vi "rsscope_core_global.vi"() -> ()   [LabVIEW 2014] (continued)
"Supported Models"="RTO|RTP", "Instrument Options"="K72", "Flags"=0, "Help"="Sets the completer ID to be searched for in the transaction layer type.\n\nAvailable Repeated Capabilities:\nNone\n\nRemote-control command(s):\nSEARch:TRIGger:PCIE:TLP:CPID"}, {"Level"=4, "Class Only"=TRUE, "Identifier"="", "Descriptive Name"="DLLP", "Data Type"=0, "Command"="", "Access"=0, "Range Table"="", "Read Callback"="", "Write Callback"="", "Supported Models"="", "Instrument Options"="", "Flags"=0, "Help"="Configures data link layer search."}, {"Level"=5, "Class Only"=FALSE, "Identifier"="RSSCOPE_ATTR_PCIE_SEARCH_DLLP", "Descriptive Name"="PCIe Search DLLP", "Data Type"=0, "Command"="SEAR:TRIG:PCIE:DLLP:TYPE", "Access"=2, "Range Table"="RsScope_rngPCIeDLLP", "Read Callback"="rsscope_FormatSearchNameInt32_ReadCallback.vi", "Write Callback"="rsscope_FormatSearchNameInt32_WriteCallback.vi", "Supported Models"="RTO|RTP", "Instrument Options"="K72", "Flags"=0, "Help"="Sets the DLLP t type to be searched for, for the data link layer.\n\nAvailable Repeated Capabilities:\nNone\n\nRemote-control command(s):\nSEARch:TRIGger:PCIE:DLLP:TYPE"}, {"Level"=5, "Class Only"=FALSE, "Identifier"="RSSCOPE_ATTR_PCIE_SEARCH_DLLP_MR_TYPE", "Descriptive Name"="PCIe Search DLLP MR Type", "Data Type"=0, "Command"="SEAR:TRIG:PCIE:DLLP:MULT:TYPE", "Access"=2, "Range Table"="RsScope_rngPCIeDLLPMRType", "Read Callback"="rsscope_FormatSearchNameInt32_ReadCallback.vi", "Write Callback"="rsscope_FormatSearchNameInt32_WriteCallback.vi", "Supported Models"="RTO|RTP", "Instrument Options"="K72", "Flags"=0, "Help"="Sets the multi-root type to be searched for, for the data link layer.\n\nAvailable Repeated Capabilities:\nNone\n\nRemote-control command(s):\nSEARch:TRIGger:PCIE:DLLP:MULT:TYPE"}, {"Level"=5, "Class Only"=FALSE, "Identifier"="RSSCOPE_ATTR_PCIE_SEARCH_DLLP_MR_INIT_PHASE", "Descriptive Name"="PCIe Search DLLP MR Init Phase", "Data Type"=0, "Command"="SEAR:TRIG:PCIE:DLLP:MULT:PHAS", "Access"=2, "Range Table"="RsScope_rngPCIeState", "Read Callback"="rsscope_FormatSearchNameInt32_ReadCallback.vi", "Write Callback"="rsscope_FormatSearchNameInt32_WriteCallback.vi", "Supported Models"="RTO|RTP", "Instrument Options"="K72", "Flags"=0, "Help"="Sets the phase state to be searched for, for the data link layer.\n\nAvailable Repeated Capabilities:\nNone\n\nRemote-control command(s):\nSEARch:TRIGger:PCIE:DLLP:MULT:PHAS"}, {"Level"=5, "Class Only"=FALSE, "Identifier"="RSSCOPE_ATTR_PCIE_SEARCH_DLLP_MR_INIT_VH_FC", "Descriptive Name"="PCIe Search DLLP MR Init VH FC", "Data Type"=0, "Command"="SEAR:TRIG:PCIE:DLLP:MULT:VHFC", "Access"=2, "Range Table"="RsScope_rngPCIeState", "Read Callback"="rsscope_FormatSearchNameInt32_ReadCallback.vi", "Write Callback"="rsscope_FormatSearchNameInt32_WriteCallback.vi", "Supported Models"="RTO|RTP", "Instrument Options"="K72", "Flags"=0, "Help"="Sets the virtual hierarchies flow control presence state to be searched for, for the data link layer.\n\nAvailable Repeated Capabilities:\nNone\n\nRemote-control command(s):\nSEARch:TRIGger:PCIE:DLLP:MULT:VHFC"}, {"Level"=5, "Class Only"=FALSE, "Identifier"="RSSCOPE_ATTR_PCIE_SEARCH_DLLP_MR_INIT_MIXED_TYPE", "Descriptive Name"="PCIe Search DLLP MR Init Mixed Type", "Data Type"=0, "Command"="SEAR:TRIG:PCIE:DLLP:MULT:MIXT", "Access"=2, "Range Table"="RsScope_rngPCIeState", "Read Callback"="rsscope_FormatSearchNameInt32_ReadCallback.vi", "Write Callback"="rsscope_FormatSearchNameInt32_WriteCallback.vi", "Supported Models"="RTO|RTP", "Instrument Options"="K72", "Flags"=0, "Help"="Sets the mixed type presence state to be searched for, for the data link layer.\n\nAvailable Repeated Capabilities:\nNone\n\nRemote-control command(s):\nSEARch:TRIGger:PCIE:DLLP:MULT:MIXT"}, {"Level"=5, "Class Only"=FALSE, "Identifier"="RSSCOPE_ATTR_PCIE_SEARCH_DLLP_MR_INIT_AUTHORIZED", "Descriptive Name"="PCIe Search DLLP MR Init Authorized", "Data Type"=0, "Command"="SEAR:TRIG:PCIE:DLLP:MULT:AUTH", "Access"=2, "Range Table"="RsScope_rngPCIeState", "Read Callback"="rsscope_FormatSearchNameInt32_ReadCallback.vi", "Write Callback"="rsscope_FormatSearchNameInt32_WriteCallback.vi", "Supported Models"="RTO|RTP", "Instrument Options"="K72", "Flags"=0, "Help"="Sets the authorized presence state to be searched for, for the data link layer.\n\nAvailable Repeated Capabilities:\nNone\n\nRemote-control command(s):\nSEARch:TRIGger:PCIE:DLLP:MULT:AUTH"}, {"Level"=5, "Class Only"=FALSE, "Identifier"="RSSCOPE_ATTR_PCIE_SEARCH_DLLP_MR_INIT_DEVICE_PORT_TYPE", "Descriptive Name"="PCIe Search DLLP MR Init Device Port Type", "Data Type"=0, "Command"="SEAR:TRIG:PCIE:DLLP:MULT:DVPT", "Access"=2, "Range Table"="RsScope_rngPCIeDevicePortType", "Read Callback"="rsscope_FormatSearchNameInt32_ReadCallback.vi", "Write Callback"="rsscope_FormatSearchNameInt32_WriteCallback.vi", "Supported Models"="RTO|RTP", "Instrument Options"="K72", "Flags"=0, "Help"="Sets the device/port type to be searched for, for the data link layer.\n\nAvailable Repeated Capabilities:\nNone\n\nRemote-control command(s):\nSEARch:TRIGger:PCIE:DLLP:MULT:DVPT"}, {"Level"=5, "Class Only"=FALSE, "Identifier"="RSSCOPE_ATTR_PCIE_SEARCH_DLLP_MR_VL_NUMBER", "Descriptive Name"="PCIe Search DLLP MR VL Number", "Data Type"=0, "Command"="SEAR:TRIG:PCIE:DLLP:MULT:VLNR", "Access"=2, "Range Table"="RsScope_rngPCIeVLNumber", "Read Callback"="rsscope_FormatSearchNameInt32_ReadCallback.vi", "Write Callback"="rsscope_FormatSearchNameInt32_WriteCallback.vi", "Supported Models"="RTO|RTP", "Instrument Options"="K72", "Flags"=0, "Help"="Sets the virtual link (VL) number to be searched for, for the data link layer.\n\nAvailable Repeated Capabilities:\nNone\n\nRemote-control command(s):\nSEARch:TRIGger:PCIE:DLLP:MULT:VLNR"}, {"Level"=5, "Class Only"=FALSE, "Identifier"="RSSCOPE_ATTR_PCIE_SEARCH_DLLP_MR_VH_ABSENT", "Descriptive Name"="PCIe Search DLLP MR VH Absent", "Data Type"=0, "Command"="SEAR:TRIG:PCIE:DLLP:MULT:HABS", "Access"=2, "Range Table"="RsScope_rngPCIeState", "Read Callback"="rsscope_FormatSearchNameInt32_ReadCallback.vi", "Write Callback"="rsscope_FormatSearchNameInt32_WriteCallback.vi", "Supported Models"="RTO|RTP", "Instrument Options"="K72", "Flags"=0, "Help"="Sets the state of the absent virtual hieararchies (VH) to be searched for, for the data link layer.\n\nAvailable Repeated Capabilities:\nNone\n\nRemote-control command(s):\nSEARch:TRIGger:PCIE:DLLP:MULT:HABS"}, {"Level"=5, "Class Only"=FALSE, "Identifier"="RSSCOPE_ATTR_PCIE_SEARCH_DLLP_MR_TLP_TYPE", "Descriptive Name"="PCIe Search DLLP MR TLP Type", "Data Type"=0, "Command"="SEAR:TRIG:PCIE:DLLP:MULT:TLPT", "Access"=2, "Range Table"="RsScope_rngPCIeDLLPMRTLPType", "Read Callback"="rsscope_FormatSearchNameInt32_ReadCallback.vi", "Write Callback"="rsscope_FormatSearchNameInt32_WriteCallback.vi", "Supported Models"="RTO|RTP", "Instrument Options"="K72", "Flags"=0, "Help"="Sets the multi-root type to be searched for, for the data link layer.\n\nAvailable Repeated Capabilities:\nNone\n\nRemote-control command(s):\nSEARch:TRIGger:PCIE:DLLP:MULT:TLPT"}, {"Level"=5, "Class Only"=FALSE, "Identifier"="RSSCOPE_ATTR_PCIE_SEARCH_DLLP_MR_CREDIT_TYPE", "Descriptive Name"="PCIe Search DLLP MR Credit Type", "Data Type"=0, "Command"="SEAR:TRIG:PCIE:DLLP:MULT:CRET", "Access"=2, "Range Table"="RsScope_rngPCIeDLLPMRCreditType", "Read Callback"="rsscope_FormatSearchNameInt32_ReadCallback.vi", "Write Callback"="rsscope_FormatSearchNameInt32_WriteCallback.vi", "Supported Models"="RTO|RTP", "Instrument Options"="", "Flags"=0, "Help"="Sets the credit type to be searched for, for the data link layer.\n\nAvailable Repeated Capabilities:\nNone\n\nRemote-control command(s):\nSEARch:TRIGger:PCIE:DLLP:MULT:CRET"}, {"Level"=5, "Class Only"=FALSE, "Identifier"="RSSCOPE_ATTR_PCIE_SEARCH_DLLP_MR_A", "Descriptive Name"="PCIe Search DLLP MR A", "Data Type"=0, "Command"="SEAR:TRIG:PCIE:DLLP:MULT:RESA", "Access"=2, "Range Table"="RsScope_rngPCIeTriggerDLLPMRA", "Read Callback"="rsscope_FormatSearchNameInt32_ReadCallback.vi", "Write Callback"="rsscope_FormatSearchNameInt32_WriteCallback.vi", "Supported Models"="RTO|RTP", "Instrument Options"="K72", "Flags"=0, "Help"="Sets the on the value of the A bit to be searched for, for the data link layer.\n\nAvailable Repeated Capabilities:\nNone\n\nRemote-control command(s):\nSEARch:TRIGger:PCIE:DLLP:MULT:RESA"}, {"Level"=5, "Class Only"=FALSE, "Identifier"="RSSCOPE_ATTR_PCIE_SEARCH_DLLP_MR_VH_GROUP", "Descriptive Name"="PCIe Search DLLP MR VH Group", "Data Type"=0, "Command"="SEAR:TRIG:PCIE:DLLP:MULT:VHGR", "Access"=2, "Range Table"="RsScope_rngPCIeDLLPVHGroup", "Read Callback"="rsscope_FormatSearchNameInt32_ReadCallback.vi", "Write Callback"="rsscope_FormatSearchNameInt32_WriteCallback.vi", "Supported Models"="RTO|RTP", "Instrument Options"="K72", "Flags"=0, "Help"="Sets the virtual hierarchies group to be searched for, for the data link layer.\n\nAvailable Repeated Capabilities:\nNone\n\nRemote-control command(s):\nSEARch:TRIGger:PCIE:DLLP:MULT:VHGR"}, {"Level"=5, "Class Only"=FALSE, "Identifier"="RSSCOPE_ATTR_PCIE_SEARCH_DLLP_SEQUENCE", "Descriptive Name"="PCIe Search DLLP Sequence", "Data Type"=2, "Command"="SEAR:TRIG:PCIE:DLLP:SEQ", "Access"=2, "Range Table"="", "Read Callback"="rsscope_FormatSearchNameString_ReadCallback.vi", "Write Callback"="rsscope_FormatSearchNameString_WriteCallback.vi", "Supported Models"="RTO|RTP", "Instrument Options"="K72", "Flags"=0, "Help"="Sets the sequence field, indicating what TLPs are affected by the ACK/NAK, to be searched for, for the data link layer.\n\nAvailable Repeated Capabilities:\nNone\n\nRemote-control command(s):\nSEARch:TRIGger:PCIE:DLLP:SEQ"}, {"Level"=5, "Class Only"=FALSE, "Identifier"="RSSCOPE_ATTR_PCIE_SEARCH_DLLP_FC_CREDIT_TYPE", "Descriptive Name"="PCIe Search DLLP FC Credit Type", "Data Type"=0, "Command"="SEAR:TRIG:PCIE:DLLP:FCTL:CRET", "Access"=2, "Range Table"="RsScope_rngPCIeDLLPFCCreditType", "Read Callback"="rsscope_FormatSearchNameInt32_ReadCallback.vi", "Write Callback"="rsscope_FormatSearchNameInt32_WriteCallback.vi", "Supported Models"="RTO|RTP", "Instrument Options"="K72", "Flags"=0, "Help"="Sets credit type value to be searched for, for the data link layer.\n\nAvailable Repeated Capabilities:\nNone\n\nRemote-control command(s):\nSEARch:TRIGger:PCIE:DLLP:FCTL:CRET"}, {"Level"=5, "Class Only"=FALSE, "Identifier"="RSSCOPE_ATTR_PCIE_SEARCH_DLLP_FC_VC_ID", "Descriptive Name"="PCIe Search DLLP FC VC ID", "Data Type"=0, "Command"="SEAR:TRIG:PCIE:DLLP:FCTL:VCID", "Access"=2, "Range Table"="RsScope_rngPCIeDLLPVCID", "Read Callback"="rsscope_FormatSearchNameInt32_ReadCallback.vi", "Write Callback"="rsscope_FormatSearchNameInt32_WriteCallback.vi", "Supported Models"="RTO|RTP", "Instrument Options"="K72", "Flags"=0, "Help"="Sets the virtual channel ID to be searched for, for the data link layer.\n\nAvailable Repeated Capabilities:\nNone\n\nRemote-control command(s):\nSEARch:TRIGger:PCIE:DLLP:FCTL:VCID"}, {"Level"=5, "Class Only"=FALSE, "Identifier"="RSSCOPE_ATTR_PCIE_SEARCH_DLLP_PM_TYPE", "Descriptive Name"="PCIe Search DLLP PM Type", "Data Type"=0, "Command"="SEAR:TRIG:PCIE:DLLP:POWM", "Access"=2, "Range Table"="RsScope_rngPCIeDLLPPMType", "Read Callback"="rsscope_FormatSearchNameInt32_ReadCallback.vi", "Write Callback"="rsscope_FormatSearchNameInt32_WriteCallback.vi", "Supported Models"="RTO|RTP", "Instrument Options"="K72", "Flags"=0, "Help"="Sets the power management type to be searched for, for the data link layer.\n\nAvailable Repeated Capabilities:\nNone\n\nRemote-control command(s):\nSEARch:TRIGger:PCIE:DLLP:POWM"}, {"Level"=5, "Class Only"=FALSE, "Identifier"="RSSCOPE_ATTR_PCIE_SEARCH_DLLP_VENDOR_PATTERN", "Descriptive Name"="PCIe Search DLLP Vendor Pattern", "Data Type"=2, "Command"="SEAR:TRIG:PCIE:DLLP:VPAT", "Access"=2, "Range Table"="", "Read Callback"="rsscope_FormatSearchNameString_ReadCallback.vi", "Write Callback"="rsscope_FormatSearchNameString_WriteCallback.vi", "Supported Models"="RTO|RTP", "Instrument Options"="K72", "Flags"=0, "Help"="Sets the vendor pattern to be searched for, for the data link layer.\n\nAvailable Repeated Capabilities:\nNone\n\nRemote-control command(s):\nSEARch:TRIGger:PCIE:DLLP:VPAT"}, {"Level"=4, "Class Only"=TRUE, "Identifier"="", "Descriptive Name"="Ordered Sets", "Data Type"=0, "Command"="", "Access"=0, "Range Table"="", "Read Callback"="", "Write Callback"="", "Supported Models"="", "Instrument Options"="", "Flags"=0, "Help"="Configures the search on a defined ordered set."}, {"Level"=5, "Class Only"=FALSE, "Identifier"="RSSCOPE_ATTR_PCIE_SEARCH_OSET_TRAINING_SEQUENCE_1", "Descriptive Name"="PCIe Search OSET Training Sequence 1", "Data Type"=3, "Command"="SEAR:TRIG:PCIE:OSET:TSON", "Access"=2, "Range Table"="", "Read Callback"="rsscope_FormatSearchNameBoolean_ReadCallback.vi", "Write Callback"="rsscope_FormatSearchNameBoolean_WriteCallback.vi", "Supported Models"="RTO|RTP", "Instrument Options"="K72", "Flags"=0, "Help"="Enables searching for training sequence 1 ordered sets.\n\nAvailable Repeated Capabilities:\nNone\n\nRemote-control command(s):\nSEARch:TRIGger:PCIE:OSET:TSONe"}, {"Level"=5, "Class Only"=FALSE, "Identifier"="RSSCOPE_ATTR_PCIE_SEARCH_OSET_TRAINING_SEQUENCE_2", "Descriptive Name"="PCIe Search OSET Training Sequence 2", "Data Type"=3, "Command"="SEARch:TRIGger:PCIE:OSET:TSTWo", "Access"=2, "Range Table"="", "Read Callback"="rsscope_FormatSearchNameBoolean_ReadCallback.vi", "Write Callback"="rsscope_FormatSearchNameBoolean_WriteCallback.vi", "Supported Models"="RTO|RTP", "Instrument Options"="K72", "Flags"=0, "Help"="Enables searching for training sequence 2 ordered sets.\n\nAvailable Repeated Capabilities:\nNone\n\nRemote-control command(s):\nSEARch:TRIGger:PCIE:OSET:TSTWo"}, {"Level"=5, "Class Only"=FALSE, "Identifier"="RSSCOPE_ATTR_PCIE_SEARCH_OSET_FAST_TRAINING_SEQUENCE", "Descriptive Name"="PCIe Search OSET Fast Training Sequence", "Data Type"=3, "Command"="SEAR:TRIG:PCIE:OSET:FTS", "Access"=2, "Range Table"="", "Read Callback"="rsscope_FormatSearchNameBoolean_ReadCallback.vi", "Write Callback"="rsscope_FormatSearchNameBoolean_WriteCallback.vi", "Supported Models"="RTO|RTP", "Instrument Options"="K72", "Flags"=0, "Help"="Enables searching for fast training sequence ordered sets.\n\nAvailable Repeated Capabilities:\nNone\n\nRemote-control command(s):\nSEARch:TRIGger:PCIE:OSET:FTS"}, {"Level"=5, "Class Only"=FALSE, "Identifier"="RSSCOPE_ATTR_PCIE_SEARCH_OSET_EIDL", "Descriptive Name"="PCIe Search OSET Electrical Idle", "Data Type"=3, "Command"="SEAR:TRIG:PCIE:OSET:EIDL", "Access"=2, "Range Table"="", "Read Callback"="rsscope_FormatSearchNameBoolean_ReadCallback.vi", "Write Callback"="rsscope_FormatSearchNameBoolean_WriteCallback.vi", "Supported Models"="RTO|RTP", "Instrument Options"="K72", "Flags"=0, "Help"="Enables searching for electrical idle ordered sets.\n\nAvailable Repeated Capabilities:\nNone\n\nRemote-control command(s):\nSEARch:TRIGger:PCIE:OSET:EIDL"}, {"Level"=5, "Class Only"=FALSE, "Identifier"="RSSCOPE_ATTR_PCIE_SEARCH_OSET_EIDE", "Descriptive Name"="PCIe Search OSET Electrical Idle Exit", "Data Type"=3, "Command"="SEAR:TRIG:PCIE:OSET:EIDE", "Access"=2, "Range Table"="", "Read Callback"="rsscope_FormatSearchNameBoolean_ReadCallback.vi", "Write Callback"="rsscope_FormatSearchNameBoolean_WriteCallback.vi", "Supported Models"="RTO|RTP", "Instrument Options"="K72", "Flags"=0, "Help"="Enables searching for electrical idle exit ordered sets.\n\nAvailable Repeated Capabilities:\nNone\n\nRemote-control command(s):\nSEARch:TRIGger:PCIE:OSET:EIDE"}, {"Level"=5, "Class Only"=FALSE, "Identifier"="RSSCOPE_ATTR_PCIE_SEARCH_OSET_SKP", "Descriptive Name"="PCIe Search OSET SKP", "Data Type"=3, "Command"="SEAR:TRIG:PCIE:OSET:SKIP", "Access"=2, "Range Table"="", "Read Callback"="rsscope_FormatSearchNameBoolean_ReadCallback.vi", "Write Callback"="rsscope_FormatSearchNameBoolean_WriteCallback.vi", "Supported Models"="RTO|RTP", "Instrument Options"="K72", "Flags"=0, "Help"="Enables searching for SKP ordered sets.\n\nAvailable Repeated Capabilities:\nNone\n\nRemote-control command(s):\nSEARch:TRIGger:PCIE:OSET:SKIP"}, {"Level"=5, "Class Only"=FALSE, "Identifier"="RSSCOPE_ATTR_PCIE_SEARCH_OSET_COMP", "Descriptive Name"="PCIe Search OSET Compliance Pattern", "Data Type"=3, "Command"="SEAR:TRIG:PCIE:OSET:COMP", "Access"=2, "Range Table"="", "Read Callback"="rsscope_FormatSearchNameBoolean_ReadCallback.vi", "Write Callback"="rsscope_FormatSearchNameBoolean_WriteCallback.vi", "Supported Models"="RTO|RTP", "Instrument Options"="K72", "Flags"=0, "Help"="Enables searching forcompliance pattern ordered sets.\n\nAvailable Repeated Capabilities:\nNone\n\nRemote-control command(s):\nSEARch:TRIGger:PCIE:OSET:COMP"}, {"Level"=5, "Class Only"=FALSE, "Identifier"="RSSCOPE_ATTR_PCIE_SEARCH_OSET_START_OF_DATA_SEQUENCE", "Descriptive Name"="PCIe Search OSET Start Of Data Sequence", "Data Type"=3, "Command"="SEAR:TRIG:PCIE:OSET:SDS", "Access"=2, "Range Table"="", "Read Callback"="rsscope_FormatSearchNameBoolean_ReadCallback.vi", "Write Callback"="rsscope_FormatSearchNameBoolean_WriteCallback.vi", "Supported Models"="RTO|RTP", "Instrument Options"="K72", "Flags"=0, "Help"="Enables searching for a start of data sequence order set.\n\nAvailable Repeated Capabilities:\nNone\n\nRemote-control command(s):\nSEARch:TRIGger:PCIE:OSET:SDS"}, {"Level"=4, "Class Only"=TRUE, "Identifier"="", "Descriptive Name"="Error Condition", "Data Type"=0, "Command"="", "Access"=0, "Range Table"="", "Read Callback"="", "Write Callback"="", "Supported Models"="", "Instrument Options"="", "Flags"=0, "Help"="Search on enabled error condition."}, {"Level"=5, "Class Only"=FALSE, "Identifier"="RSSCOPE_ATTR_PCIE_SEARCH_ERRC_CRC16", "Descriptive Name"="PCIe Search ERRC CRC16 Error", "Data Type"=3, "Command"="SEAR:TRIG:PCIE:ERRC:CRC", "Access"=2, "Range Table"="", "Read Callback"="rsscope_FormatSearchNameBoolean_ReadCallback.vi", "Write Callback"="rsscope_FormatSearchNameBoolean_WriteCallback.vi", "Supported Models"="RTO|RTP", "Instrument Options"="K72", "Flags"=0, "Help"="Enables searching for 16-bit cyclic redundancy check (CRC) errors.\n\nAvailable Repeated Capabilities:\nNone\n\nRemote-control command(s):\nSEARch:TRIGger:PCIE:ERRC:CRC"}, {"Level"=5, "Class Only"=FALSE, "Identifier"="RSSCOPE_ATTR_PCIE_SEARCH_ERRC_LCRC", "Descriptive Name"="PCIe Search ERRC LCRC Error", "Data Type"=3, "Command"="SEAR:TRIG:PCIE:ERRC:LCRC", "Access"=2, "Range Table"="", "Read Callback"="rsscope_FormatSearchNameBoolean_ReadCallback.vi", "Write Callback"="rsscope_FormatSearchNameBoolean_WriteCallback.vi", "Supported Models"="RTO|RTP", "Instrument Options"="K72", "Flags"=0, "Help"="Enables searching for link cyclic redundancy check (LCRC) errors.\n\nAvailable Repeated Capabilities:\nNone\n\nRemote-control command(s):\nSEARch:TRIGger:PCIE:ERRC:LCRC"}, {"Level"=5, "Class Only"=FALSE, "Identifier"="RSSCOPE_ATTR_PCIE_SEARCH_ERRC_ECRC", "Descriptive Name"="PCIe Search ERRC ECRC Error", "Data Type"=3, "Command"="SEAR:TRIG:PCIE:ERRC:ECRC", "Access"=2, "Range Table"="", "Read Callback"="rsscope_FormatSearchNameBoolean_ReadCallback.vi", "Write Callback"="rsscope_FormatSearchNameBoolean_WriteCallback.vi", "Supported Models"="RTO|RTP", "Instrument Options"="K72", "Flags"=0, "Help"="Enables searching for end-to-end cyclic redundancy checksum (ECRC) errors.\n\nAvailable Repeated Capabilities:\nNone\n\nRemote-control command(s):\nSEARch:TRIGger:PCIE:ERRC:ECRC"}, {"Level"=5, "Class Only"=FALSE, "Identifier"="RSSCOPE_ATTR_PCIE_SEARCH_ERRC_INVALID_SYMBOL", "Descriptive Name"="PCIe Search ERRC Invalid Symbol", "Data Type"=3, "Command"="SEAR:TRIG:PCIE:ERRC:INVP", "Access"=2, "Range Table"="", "Read Callback"="rsscope_FormatSearchNameBoolean_ReadCallback.vi", "Write Callback"="rsscope_FormatSearchNameBoolean_WriteCallback.vi", "Supported Models"="RTO|RTP", "Instrument Options"="K72", "Flags"=0, "Help"="Enables searching for invalid symbol errors.\n\nAvailable Repeated Capabilities:\nNone\n\nRemote-control command(s):\nSEARch:TRIGger:PCIE:ERRC:INVP"}, {"Level"=5, "Class Only"=FALSE, "Identifier"="RSSCOPE_ATTR_PCIE_SEARCH_ERRC_DISP", "Descriptive Name"="PCIe Search ERRC Disparity Error", "Data Type"=3, "Command"="SEAR:TRIG:PCIE:ERRC:DISP", "Access"=2, "Range Table"="", "Read Callback"="rsscope_FormatSearchNameBoolean_ReadCallback.vi", "Write Callback"="rsscope_FormatSearchNameBoolean_WriteCallback.vi", "Supported Models"="RTO|RTP", "Instrument Options"="K72", "Flags"=0, "Help"="Enables searching for disparity errors.\n\nAvailable Repeated Capabilities:\nNone\n\nRemote-control command(s):\nSEARch:TRIGger:PCIE:ERRC:DISP"}, {"Level"=5, "Class Only"=FALSE, "Identifier"="RSSCOPE_ATTR_PCIE_SEARCH_ERRC_LENGTH_ERROR", "Descriptive Name"="PCIe Search ERRC Length Error", "Data Type"=3, "Command"="SEAR:TRIG:PCIE:ERRC:LENG", "Access"=2, "Range Table"="", "Read Callback"="rsscope_FormatSearchNameBoolean_ReadCallback.vi", "Write Callback"="rsscope_FormatSearchNameBoolean_WriteCallback.vi", "Supported Models"="RTO|RTP", "Instrument Options"="K72", "Flags"=0, "Help"="Enables searching for length error.\n\nAvailable Repeated Capabilities:\nNone\n\nRemote-control command(s):\nSEARch:TRIGger:PCIE:ERRC:LENGth"}, {"Level"=5, "Class Only"=FALSE, "Identifier"="RSSCOPE_ATTR_PCIE_SEARCH_ERRC_MALFORMED_ERROR", "Descriptive Name"="PCIe Search ERRC Malformed Error", "Data Type"=3, "Command"="SEAR:TRIG:PCIE:ERRC:MALF", "Access"=2, "Range Table"="", "Read Callback"="rsscope_FormatSearchNameBoolean_ReadCallback.vi", "Write Callback"="rsscope_FormatSearchNameBoolean_WriteCallback.vi", "Supported Models"="RTO|RTP", "Instrument Options"="K72", "Flags"=0, "Help"="Searches for a malformed TLP: a TLP that violates specific TLP formation rules that are defined in the specification.\n\nAvailable Repeated Capabilities:\nNone\n\nRemote-control command(s):\nSEARch:TRIGger:PCIE:ERRC:MALFormed"}, {"Level"=5, "Class Only"=FALSE, "Identifier"="RSSCOPE_ATTR_PCIE_SEARCH_ERRC_MAX_END_PREFIX", "Descriptive Name"="PCIe Search ERRC Max End Prefix", "Data Type"=3, "Command"="SEAR:TRIG:PCIE:ERRC:MXPF", "Access"=2, "Range Table"="", "Read Callback"="rsscope_FormatSearchNameBoolean_ReadCallback.vi", "Write Callback"="rsscope_FormatSearchNameBoolean_WriteCallback.vi", "Supported Models"="RTO|RTP", "Instrument Options"="K72", "Flags"=0, "Help"="Enables searching for an end-end prefix error. The maximum number of permitted end-end TLP prefixes is 4.\n\nAvailable Repeated Capabilities:\nNone\n\nRemote-control command(s):\nSEARch:TRIGger:PCIE:ERRC:MXPFix"}, {"Level"=5, "Class Only"=FALSE, "Identifier"="RSSCOPE_ATTR_PCIE_SEARCH_ERRC_PREFIX_ORDER_ERROR", "Descriptive Name"="PCIe Search ERRC Prefix Order Error", "Data Type"=3, "Command"="SEAR:TRIG:PCIE:ERRC:PFOR", "Access"=2, "Range Table"="", "Read Callback"="rsscope_FormatSearchNameBoolean_ReadCallback.vi", "Write Callback"="rsscope_FormatSearchNameBoolean_WriteCallback.vi", "Supported Models"="RTO|RTP", "Instrument Options"="K72", "Flags"=0, "Help"="Enables searching for a wrong prefix order\n\nAvailable Repeated Capabilities:\nNone\n\nRemote-control command(s):\nSEARch:TRIGger:PCIE:ERRC:PFORder"}, {"Level"=5, "Class Only"=FALSE, "Identifier"="RSSCOPE_ATTR_PCIE_SEARCH_ERRC_SYNC_BIT", "Descriptive Name"="PCIe Search ERRC Sync Bit", "Data Type"=3, "Command"="SEAR:TRIG:PCIE:ERRC:SYCB", "Access"=2, "Range Table"="", "Read Callback"="rsscope_FormatSearchNameBoolean_ReadCallback.vi", "Write Callback"="rsscope_FormatSearchNameBoolean_WriteCallback.vi", "Supported Models"="RTO|RTP", "Instrument Options"="K72", "Flags"=0, "Help"="Enables searching for a sync bit\n\nAvailable Repeated Capabilities:\nNone\n\nRemote-control command(s):\nSEARch:TRIGger:PCIE:ERRC:SYCBit"}, {"Level"=5, "Class Only"=FALSE, "Identifier"="RSSCOPE_ATTR_PCIE_SEARCH_ERRC_UNKNOWN_PACKET", "Descriptive Name"="PCIe Search ERRC Unknown Packet", "Data Type"=3, "Command"="SEAR:TRIG:PCIE:ERRC:UKNP", "Access"=2, "Range Table"="", "Read Callback"="rsscope_FormatSearchNameBoolean_ReadCallback.vi", "Write Callback"="rsscope_FormatSearchNameBoolean_WriteCallback.vi", "Supported Models"="RTO|RTP", "Instrument Options"="K72", "Flags"=0, "Help"="Enables searching for an unknown packet.\n\nAvailable Repeated Capabilities:\nNone\n\nRemote-control command(s):\nSEARch:TRIGger:PCIE:ERRC:UKNP"}, {"Level"=5, "Class Only"=FALSE, "Identifier"="RSSCOPE_ATTR_PCIE_SEARCH_ERRC_VALUE_OUT_OF_RANGE", "Descriptive Name"="PCIe Search ERRC Value Out Of Range", "Data Type"=3, "Command"="SEAR:TRIG:PCIE:ERRC:VOOR", "Access"=2, "Range Table"="", "Read Callback"="rsscope_FormatSearchNameBoolean_ReadCallback.vi", "Write Callback"="rsscope_FormatSearchNameBoolean_WriteCallback.vi", "Supported Models"="RTO|RTP", "Instrument Options"="K72", "Flags"=0, "Help"="Triggers, if a value is out of range.\n\nAvailable Repeated Capabilities:\nNone\n\nRemote-control command(s):\nSEARch:TRIGger:PCIE:ERRC:VOORange"}, {"Level"=4, "Class Only"=TRUE, "Identifier"="", "Descriptive Name"="Results", "Data Type"=0, "Command"="", "Access"=0, "Range Table"="", "Read Callback"="", "Write Callback"="", "Supported Models"="", "Instrument Options"="", "Flags"=0, "Help"="Searches the PCIe decoding results."}, {"Level"=5, "Class Only"=FALSE, "Identifier"="RSSCOPE_ATTR_SEARCH_PCIE_PACKET_COUNT", "Descriptive Name"="Search PCIe Packet Count", "Data Type"=0, "Command"="SEAR:RES:PCIE:PCO?", "Access"=0, "Range Table"="", "Read Callback"="rsscope_FormatSearchNameInt32_ReadCallback.vi", "Write Callback"="", "Supported Models"="RTO|RTP", "Instrument Options"="K72", "Flags"=0, "Help"="Returns the packet count for the selected serial bus, i.e. the number of packets in the present acquisition.\n\nAvailable Repeated Capabilities:\nNone\n\nRemote-control command(s):\nSEARch:RESult:PCIE:PCOunt?"}, {"Level"=3, "Class Only"=TRUE, "Identifier"="", "Descriptive Name"="DDR", "Data Type"=0, "Command"="", "Access"=0, "Range Table"="", "Read Callback"="", "Write Callback"="", "Supported Models"="", "Instrument Options"="", "Flags"=0, "Help"="Configures DDR search"}, {"Level"=4, "Class Only"=TRUE, "Identifier"="", "Descriptive Name"="Results", "Data Type"=0, "Command"="", "Access"=0, "Range Table"="", "Read Callback"="", "Write Callback"="", "Supported Models"="", "Instrument Options"="", "Flags"=0, "Help"="Returns the search results."}, {"Level"=5, "Class Only"=FALSE, "Identifier"="RSSCOPE_ATTR_SEARCH_DDR_FRAME_COUNT", "Descriptive Name"="Search DDR Frame Count", "Data Type"=0, "Command"="SEAR:RES:DDR:FCO?", "Access"=0, "Range Table"="", "Read Callback"="rsscope_FormatSearchNameInt32_ReadCallback.vi", "Write Callback"="", "Supported Models"="", "Instrument Options"="K91|K93", "Flags"=0, "Help"="Returns the number of decoded frames in the search result.\n\nAvailable Repeated Capabilities:\nNone\n\nRemote-control command(s):\nSEARch:RESult:DDR:FCOunt?"}, {"Level"=3, "Class Only"=TRUE, "Identifier"="", "Descriptive Name"="100BASE-T1", "Data Type"=0, "Command"="", "Access"=0, "Range Table"="", "Read Callback"="", "Write Callback"="", "Supported Models"="", "Instrument Options"="", "Flags"=0, "Help"="Configures 100BASE-T1 search"}, {"Level"=4, "Class Only"=FALSE, "Identifier"="RSSCOPE_ATTR_SEARCH_100BASE_T1_TYPE", "Descriptive Name"="Search 100BASE-T1 Type", "Data Type"=0, "Command"="SEAR:TRIG:HBTO:TYPE", "Access"=2, "Range Table"="RsScope_rng100BASE_T1FrameType", "Read Callback"="rsscope_FormatSearchNameInt32_ReadCallback.vi", "Write Callback"="rsscope_FormatSearchNameInt32_WriteCallback.vi", "Supported Models"="", "Instrument Options"="K57", "Flags"=0, "Help"="Selects the type of frame to be searched for.\n\nAvailable Repeated Capabilities:\nNone\n\nRemote-control command(s):\nSEARch:TRIGger:HBTO:TYPE"}, {"Level"=4, "Class Only"=FALSE, "Identifier"="RSSCOPE_ATTR_SEARCH_100BASE_T1_DESTINATION_ADDRESS_CONDITION", "Descriptive Name"="Search 100BASE-T1 Destination Address Condition", "Data Type"=0, "Command"="SEAR:TRIG:HBTO:DADD:COND", "Access"=2, "Range Table"="rsscope_rngProtocolTriggerCondition", "Read Callback"="rsscope_FormatSearchNameInt32_ReadCallback.vi", "Write Callback"="rsscope_FormatSearchNameInt32_WriteCallback.vi", "Supported Models"="", "Instrument Options"="K57", "Flags"=0, "Help"="Sets the condition for the destination address. You can define an exact value or a value range.\n\nAvailable Repeated Capabilities:\nNone\n\nRemote-control command(s):\nSEARch:TRIGger:HBTO:DADDress:CONDition"}, {"Level"=4, "Class Only"=FALSE, "Identifier"="RSSCOPE_ATTR_SEARCH_100BASE_T1_DESTINATION_ADDRESS_MAX", "Descriptive Name"="Search 100BASE-T1 Destination Address Max", "Data Type"=2, "Command"="SEAR:TRIG:HBTO:DADD:MAX", "Access"=2, "Range Table"="", "Read Callback"="rsscope_FormatSearchNameString_ReadCallback.vi", "Write Callback"="rsscope_FormatSearchNameString_WriteCallback.vi", "Supported Models"="", "Instrument Options"="K57", "Flags"=0, "Help"="Sets the end value of the destination address range if the corresponding condition is set to In Range or Out Of Range.\n\nAvailable Repeated Capabilities:\nNone\n\nRemote-control command(s):\nSEARch:TRIGger:HBTO:DADDress:MAX"}, {"Level"=4, "Class Only"=FALSE, "Identifier"="RSSCOPE_ATTR_SEARCH_100BASE_T1_DESTINATION_ADDRESS_MIN", "Descriptive Name"="Search 100BASE-T1 Destination Address Min", "Data Type"=2, "Command"="SEAR:TRIG:HBTO:DADD:MIN", "Access"=2, "Range Table"="", "Read Callback"="rsscope_FormatSearchNameString_ReadCallback.vi", "Write Callback"="rsscope_FormatSearchNameString_WriteCallback.vi", "Supported Models"="", "Instrument Options"="K57", "Flags"=0, "Help"="Specifies the destination address bit pattern, or sets the start value of a pattern range.\n\nAvailable Repeated Capabilities:\nNone\n\nRemote-control command(s):\nSEARch:TRIGger:HBTO:DADDress:MIN"}, {"Level"=4, "Class Only"=FALSE, "Identifier"="RSSCOPE_ATTR_SEARCH_100BASE_T1_SOURCE_ADDRESS_CONDITION", "Descriptive Name"="Search 100BASE-T1 Source Address Condition", "Data Type"=0, "Command"="SEAR:TRIG:HBTO:SADD:COND", "Access"=2, "Range Table"="rsscope_rngProtocolTriggerCondition", "Read Callback"="rsscope_FormatSearchNameInt32_ReadCallback.vi", "Write Callback"="rsscope_FormatSearchNameInt32_WriteCallback.vi", "Supported Models"="", "Instrument Options"="K57", "Flags"=0, "Help"="Sets the condition for the source address. You can define an exact value or a value range.\n\nAvailable Repeated Capabilities:\nNone\n\nRemote-control command(s):\nSEARch:TRIGger:HBTO:SADDress:CONDition"}, {"Level"=4, "Class Only"=FALSE, "Identifier"="RSSCOPE_ATTR_SEARCH_100BASE_T1_SOURCE_ADDRESS_MAX", "Descriptive Name"="Search 100BASE-T1 Source Address Max", "Data Type"=2, "Command"="SEAR:TRIG:HBTO:SADD:MAX", "Access"=2, "Range Table"="", "Read Callback"="rsscope_FormatSearchNameString_ReadCallback.vi", "Write Callback"="rsscope_FormatSearchNameString_WriteCallback.vi", "Supported Models"="", "Instrument Options"="K57", "Flags"=0, "Help"="Sets the end value of the source address range if the corresponding condition is set to In Range or Out Of Range.\n\nAvailable Repeated Capabilities:\nNone\n\nRemote-control command(s):\nSEARch:TRIGger:HBTO:SADDress:MAX"}, {"Level"=4, "Class Only"=FALSE, "Identifier"="RSSCOPE_ATTR_SEARCH_100BASE_T1_SOURCE_ADDRESS_MIN", "Descriptive Name"="Search 100BASE-T1 Source Address Min", "Data Type"=2, "Command"="SEAR:TRIG:HBTO:SADD:MIN", "Access"=2, "Range Table"="", "Read Callback"="rsscope_FormatSearchNameString_ReadCallback.vi", "Write Callback"="rsscope_FormatSearchNameString_WriteCallback.vi", "Supported Models"="", "Instrument Options"="K57", "Flags"=0, "Help"="Specifies the source address bit pattern, or sets the start value of a pattern range.\n\nAvailable Repeated Capabilities:\nNone\n\nRemote-control command(s):\nSEARch:TRIGger:HBTO:SADDress:MIN"}, {"Level"=4, "Class Only"=FALSE, "Identifier"="RSSCOPE_ATTR_SEARCH_100BASE_T1_TYPE_LENGTH_CONDITION", "Descriptive Name"="Search 100BASE-T1 Type Length Condition", "Data Type"=0, "Command"="SEAR:TRIG:HBTO:LENG:COND", "Access"=2, "Range Table"="rsscope_rngProtocolTriggerCondition", "Read Callback"="rsscope_FormatSearchNameInt32_ReadCallback.vi", "Write Callback"="rsscope_FormatSearchNameInt32_WriteCallback.vi", "Supported Models"="", "Instrument Options"="K57", "Flags"=0, "Help"="Sets the condition for the length / type. You can define an exact value or a value range.\n\nAvailable Repeated Capabilities:\nNone\n\nRemote-control command(s):\nSEARch:TRIGger:HBTO:LENGth:CONDition"}, {"Level"=4, "Class Only"=FALSE, "Identifier"="RSSCOPE_ATTR_SEARCH_100BASE_T1_TYPE_LENGTH_MAX", "Descriptive Name"="Search 100BASE-T1 Type Length Max", "Data Type"=2, "Command"="SEAR:TRIG:HBTO:LENG:MAX", "Access"=2, "Range Table"="", "Read Callback"="rsscope_FormatSearchNameString_ReadCallback.vi", "Write Callback"="rsscope_FormatSearchNameString_WriteCallback.vi", "Supported Models"="", "Instrument Options"="K57", "Flags"=0, "Help"="Sets the end value of the length / type range if the corresponding condition is set to In Range or Out Of Range.\n\nAvailable Repeated Capabilities:\nNone\n\nRemote-control command(s):\nSEARch:TRIGger:HBTO:LENGth:MAX"}, {"Level"=4, "Class Only"=FALSE, "Identifier"="RSSCOPE_ATTR_SEARCH_100BASE_T1_TYPE_LENGTH_MIN", "Descriptive Name"="Search 100BASE-T1 Type Length Min", "Data Type"=2, "Command"="SEAR:TRIG:HBTO:LENG:MIN", "Access"=2, "Range Table"="", "Read Callback"="rsscope_FormatSearchNameString_ReadCallback.vi", "Write Callback"="rsscope_FormatSearchNameString_WriteCallback.vi", "Supported Models"="", "Instrument Options"="K57", "Flags"=0, "Help"="Specifies the length / type bit pattern, or sets the start value of a pattern range.\n\nAvailable Repeated Capabilities:\nNone\n\nRemote-control command(s):\nSEARch:TRIGger:HBTO:LENGth:MIN"}, {"Level"=4, "Class Only"=FALSE, "Identifier"="RSSCOPE_ATTR_SEARCH_100BASE_T1_CRC_CONDITION", "Descriptive Name"="Search 100BASE-T1 CRC Condition", "Data Type"=0, "Command"="SEAR:TRIG:HBTO:CRC:COND", "Access"=2, "Range Table"="rsscope_rngProtocolTriggerCondition", "Read Callback"="rsscope_FormatSearchNameInt32_ReadCallback.vi", "Write Callback"="rsscope_FormatSearchNameInt32_WriteCallback.vi", "Supported Models"="", "Instrument Options"="K57", "Flags"=0, "Help"="Sets the condition for the frame check. You can define an exact value or a value range.\n\nAvailable Repeated Capabilities:\nNone\n\nRemote-control command(s):\nSEARch:TRIGger:HBTO:CRC:CONDition"}, {"Level"=4, "Class Only"=FALSE, "Identifier"="RSSCOPE_ATTR_SEARCH_100BASE_T1_CRC_MAX", "Descriptive Name"="Search 100BASE-T1 CRC Max", "Data Type"=2, "Command"="SEAR:TRIG:HBTO:CRC:MAX", "Access"=2, "Range Table"="", "Read Callback"="rsscope_FormatSearchNameString_ReadCallback.vi", "Write Callback"="rsscope_FormatSearchNameString_WriteCallback.vi", "Supported Models"="", "Instrument Options"="K57", "Flags"=0, "Help"="Sets the end value of the frame check range if the corresponding condition is set to In Range or Out Of Range.\n\nAvailable Repeated Capabilities:\nNone\n\nRemote-control command(s):\nSEARch:TRIGger:HBTO:CRC:MAX"}, {"Level"=4, "Class Only"=FALSE, "Identifier"="RSSCOPE_ATTR_SEARCH_100BASE_T1_CRC_MIN", "Descriptive Name"="Search 100BASE-T1 CRC Min", "Data Type"=2, "Command"="SEAR:TRIG:HBTO:CRC:MIN", "Access"=2, "Range Table"="", "Read Callback"="rsscope_FormatSearchNameString_ReadCallback.vi", "Write Callback"="rsscope_FormatSearchNameString_WriteCallback.vi", "Supported Models"="", "Instrument Options"="K57", "Flags"=0, "Help"="Specifies the frame check bit pattern, or sets the start value of a pattern range.\n\nAvailable Repeated Capabilities:\nNone\n\nRemote-control command(s):\nSEARch:TRIGger:HBTO:CRC:MIN"}, {"Level"=4, "Class Only"=FALSE, "Identifier"="RSSCOPE_ATTR_SEARCH_100BASE_T1_DATA_CONDITION", "Descriptive Name"="Search 100BASE-T1 Data Condition", "Data Type"=0, "Command"="SEAR:TRIG:HBTO:DATA:DCON", "Access"=2, "Range Table"="rsscope_rngProtocolTriggerCondition", "Read Callback"="rsscope_FormatSearchNameInt32_ReadCallback.vi", "Write Callback"="rsscope_FormatSearchNameInt32_WriteCallback.vi", "Supported Models"="", "Instrument Options"="K57", "Flags"=0, "Help"="Sets the condition for the data. You can define an exact value or a value range.\n\nAvailable Repeated Capabilities:\nNone\n\nRemote-control command(s):\nSEARch:TRIGger:HBTO:DATA:DCONdition"}, {"Level"=4, "Class Only"=FALSE, "Identifier"="RSSCOPE_ATTR_SEARCH_100BASE_T1_DATA_MAX", "Descriptive Name"="Search 100BASE-T1 Data Max", "Data Type"=2, "Command"="SEAR:TRIG:HBTO:DATA:DMAX", "Access"=2, "Range Table"="", "Read Callback"="rsscope_FormatSearchNameString_ReadCallback.vi", "Write Callback"="rsscope_FormatSearchNameString_WriteCallback.vi", "Supported Models"="", "Instrument Options"="K57", "Flags"=0, "Help"="Sets the end value of the data range if the corresponding condition is set to In Range or Out Of Range.\n\nAvailable Repeated Capabilities:\nNone\n\nRemote-control command(s):\nSEARch:TRIGger:HBTO:DATA:DMAX"}, {"Level"=4, "Class Only"=FALSE, "Identifier"="RSSCOPE_ATTR_SEARCH_100BASE_T1_DATA_MIN", "Descriptive Name"="Search 100BASE-T1 Data Min", "Data Type"=2, "Command"="SEAR:TRIG:HBTO:DATA:DMIN", "Access"=2, "Range Table"="", "Read Callback"="rsscope_FormatSearchNameString_ReadCallback.vi", "Write Callback"="rsscope_FormatSearchNameString_WriteCallback.vi", "Supported Models"="", "Instrument Options"="K57", "Flags"=0, "Help"="Specifies the data bit pattern, or sets the start value of a pattern range.\n\nAvailable Repeated Capabilities:\nNone\n\nRemote-control command(s):\nSEARch:TRIGger:HBTO:DATA:DMIN"}, {"Level"=4, "Class Only"=FALSE, "Identifier"="RSSCOPE_ATTR_SEARCH_100BASE_T1_INDEX_CONDITION", "Descriptive Name"="Search 100BASE-T1 Index Condition", "Data Type"=0, "Command"="SEAR:TRIG:HBTO:DATA:ICON", "Access"=2, "Range Table"="rsscope_rngProtocolTriggerCondition", "Read Callback"="rsscope_FormatSearchNameInt32_ReadCallback.vi", "Write Callback"="rsscope_FormatSearchNameInt32_WriteCallback.vi", "Supported Models"="", "Instrument Options"="K57", "Flags"=0, "Help"="Sets the condition for the index. You can define an exact value or a value range.\n\nAvailable Repeated Capabilities:\nNone\n\nRemote-control command(s):\nSEARch:TRIGger:HBTO:DATA:ICONdition"}, {"Level"=4, "Class Only"=FALSE, "Identifier"="RSSCOPE_ATTR_SEARCH_100BASE_T1_INDEX_MAX", "Descriptive Name"="Search 100BASE-T1 Index Max", "Data Type"=0, "Command"="SEAR:TRIG:HBTO:DATA:IMAX", "Access"=2, "Range Table"="", "Read Callback"="rsscope_FormatSearchNameInt32_ReadCallback.vi", "Write Callback"="rsscope_FormatSearchNameInt32_WriteCallback.vi", "Supported Models"="", "Instrument Options"="K57", "Flags"=0, "Help"="Sets the end value of the index range if the corresponding condition is set to In Range or Out Of Range.\n\nAvailable Repeated Capabilities:\nNone\n\nRemote-control command(s):\nSEARch:TRIGger:HBTO:DATA:IMAX"}, {"Level"=4, "Class Only"=FALSE, "Identifier"="RSSCOPE_ATTR_SEARCH_100BASE_T1_INDEX_MIN", "Descriptive Name"="Search 100BASE-T1 Index Min", "Data Type"=0, "Command"="SEAR:TRIG:HBTO:DATA:IMIN", "Access"=2, "Range Table"="", "Read Callback"="rsscope_FormatSearchNameInt32_ReadCallback.vi", "Write Callback"="rsscope_FormatSearchNameInt32_WriteCallback.vi", "Supported Models"="", "Instrument Options"="K57", "Flags"=0, "Help"="Specifies the index bit pattern, or sets the start value of a pattern range.\n\nAvailable Repeated Capabilities:\nNone\n\nRemote-control command(s):\nSEARch:TRIGger:HBTO:DATA:IMIN"}, {"Level"=4, "Class Only"=FALSE, "Identifier"="RSSCOPE_ATTR_SEARCH_100BASE_T1_ERROR_PREAMBLE", "Descriptive Name"="Search 100BASE-T1 Error Preamble", "Data Type"=3, "Command"="SEAR:TRIG:HBTO:ERR:PRE", "Access"=2, "Range Table"="", "Read Callback"="rsscope_FormatSearchNameBoolean_ReadCallback.vi", "Write Callback"="rsscope_FormatSearchNameBoolean_WriteCallback.vi", "Supported Models"="", "Instrument Options"="K57", "Flags"=0, "Help"="Enables / disables search for preamble error.\n\nAvailable Repeated Capabilities:\n
